vi "OCR_Determine Frame type.vi"(8 "Error":errorcluster, 11 "2D Image":T1) -> (0 "Error Out":errorcluster, 2 "Frame Out":T2, 3 "Border Color Out":u32(colorbox))   [LabVIEW 2009]
uses:
  Controls/Enum/ENUM_Frame Template Select.ctl
  Controls/Array/Color Box Array_2D Icon Viewer.ctl
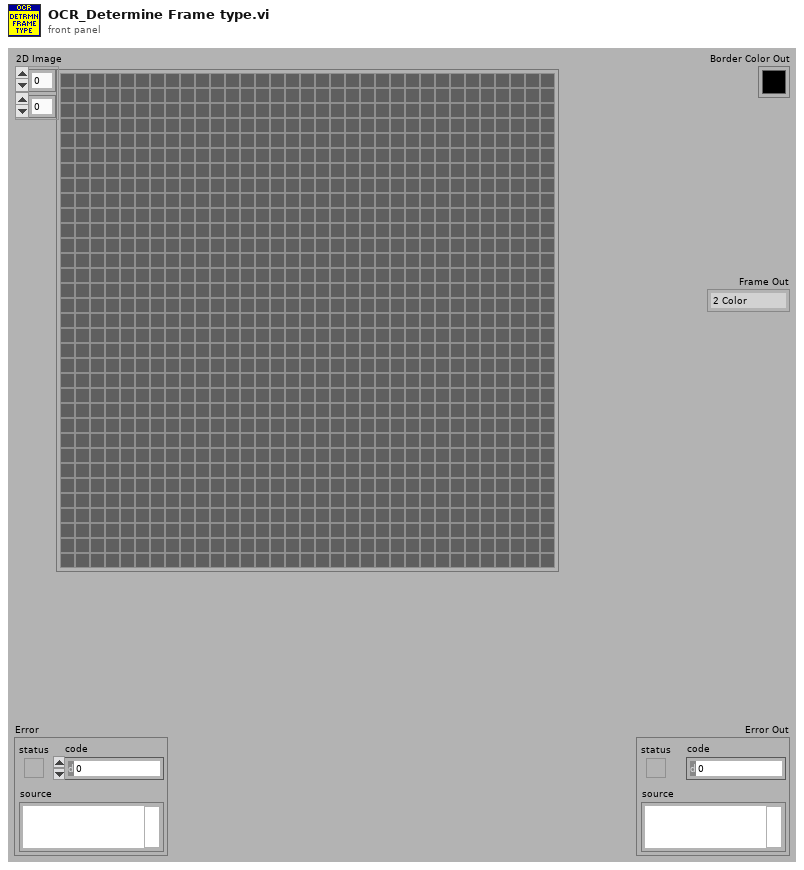
[diagram p1: front panel]
types:
  T1 = typedef "Color Box Array_2D Icon Viewer.ctl" = u32[][]
  T2 = typedef "ENUM_Frame Template Select.ctl" = enum16{"2 Color", "5 Color"}
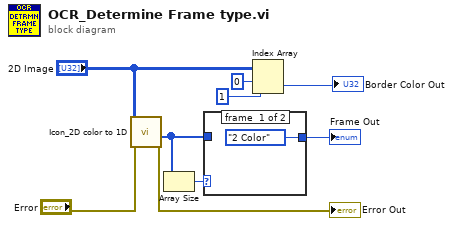
[diagram p0: block diagram]
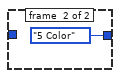
[diagram p2: hidden frame]
diagram:
  n1 = call "Icon_2D color to 1D.vi"("Error"="Error", "2D Image"="2D Image") -> ("Error Out"=→"Error Out":errorcluster, "Sorted By Quantity Out"=w7:u32[])  [unwired: 7 in, 1 out]
  n2 = Array Size(array=w7) -> (size(s)=w6:i32)
  n3 = case shown="3.." w6 {
    tunnel: w7 -> [_ _]
    tunnel: [ENUM_Frame_Template_Select."2 Color" ("Frame Out") ENUM_Frame_Template_Select."5 Color" ("Frame Out")] -> w8
    frame #0 {
    }
    frame #1 {
    }
  }
  "Frame Out" <- w8
  n4 = Index Array(array="2D Image", index (row)=0 ("index"), index (col)=1 ("disabled index (col)")) -> (element=→"Border Color Out":u32)
